vi "SoundGeneratorAD.vi"() -> ()   [LabVIEW 2019]
uses:
  <vilib>/sound2/lvsound2.llb/Sampling Mode.ctl
  <vilib>/sound2/lvsound2.llb/Sound Output Set Volume (Single).vi
  <vilib>/sound2/lvsound2.llb/Sound Output Write (DBL).vi
  <vilib>/measure/NI_MABase.lvlib
panel:
  in  "Stop":bool
  in  "Frequency Right":dbl(slide) scale=0.0..100.0
  in  "Amplitude Right":dbl(slide) scale=0.0..100.0
  in  "Frequency Left":dbl(slide) scale=0.0..100.0
  in  "Amplitude Left":dbl(slide) scale=0.0..100.0
  in  "# of samples":dbl
  in  "# of samples / ch":dbl
  in  "Volume":dbl(slide) scale=0.0..100.0
  in  "Output Device ID":dbl
  in  "Sound format":T1
  # "Default configurations for Sount format:\n\nSample rate: 44100 (Hz)\n# of channels: 2\nBits per sample: 16"
  # "How fast the sound\nis sampled per\nchannel"
  # "How fast the sound is sampled"
  # "Default: 0"
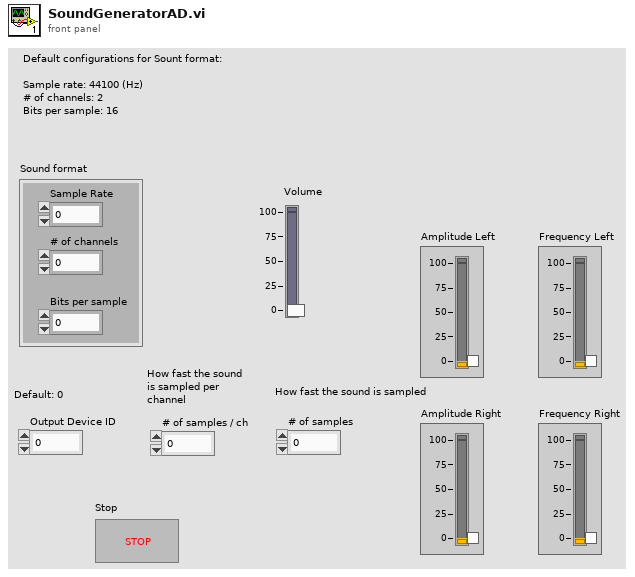
[diagram p1: front panel]
types:
  T1 = cluster{"Sample Rate":dbl, "# of channels":dbl, "Bits per sample":dbl}
  T2 = typedef "Sampling Mode.ctl" = i32
  T3 = typedef "Sound Output Task ID.ctl" = u32
  T4 = cluster{"# of samples / ch":dbl, "# of samples":dbl}
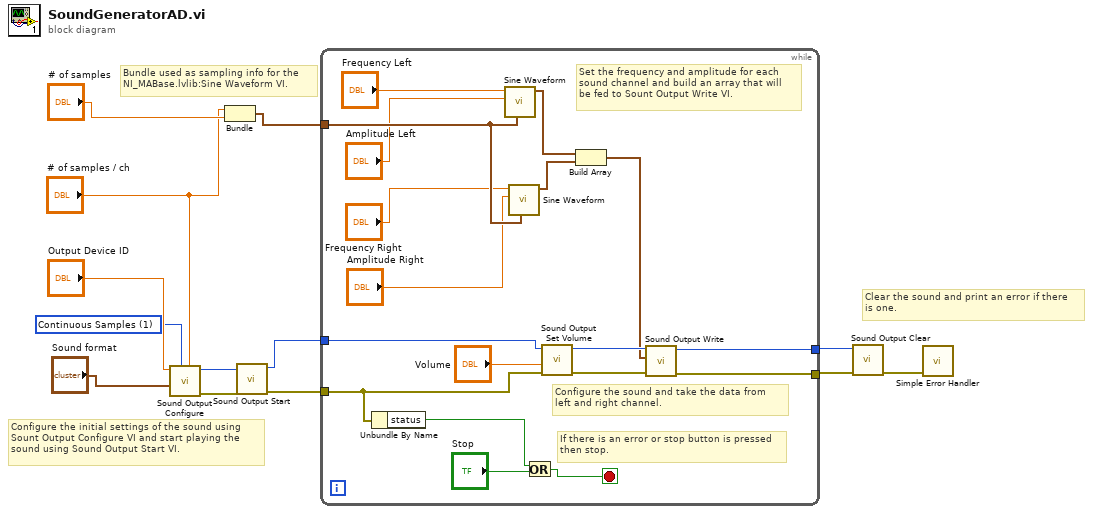
[diagram p0: block diagram]
diagram:
  w11 = T2 1 items=["Finite Samples", "Continuous Samples"] ("sample mode")
  # "Clear the sound and print an error if there\nis one."
  # "Bundle used as sampling info for the\nNI_MABase.lvlib:Sine Waveform VI."
  # "Configure the initial settings of the sound using\nSount Output Configure VI and start playing the\nsound using Sound Output Start VI."
  n1 = call <vilib>:"Sound Output Configure.vi"("number of samples/ch"="# of samples / ch", "sample mode"=w11, "sound format"="Sound format", "device ID"="Output Device ID") -> ("error out"=w10:errorcluster, "task ID"=w9:T3)  [unwired: 6 in]
  n2 = Bundle("# of samples / ch"="# of samples / ch", "# of samples"="# of samples") -> (w1:T4)  [unwired: 1 in]
  n3 = call <vilib>:"Sound Output Start.vi"("error in (no error)"=w10, "task ID"=w9) -> ("error out"=w6:errorcluster, "task ID out"=w5:T3)  [unwired: 8 in]
  n4 = while {
    tunnel: w6 -> [w28]
    tunnel: w5 -> [w26]
    tunnel: [w23] -> w4
    tunnel: [w22] -> w3
    tunnel: w1 -> [w21]
    stop <- w31 stop-if-true
    # "Set the frequency and amplitude for each\nsound channel and build an array that will\nbe fed to Sount Output Write VI."
    # "Configure the sound and take the data from\nleft and right channel."
    # "If there is an error or stop button is pressed\nthen stop."
    n5 = Unbundle By Name(w28) -> ("status"=w27:bool)
    n6 = call <vilib>:"Sine Waveform.vi"("sampling info"=w21, "amplitude"="Amplitude Left", "frequency"="Frequency Left") -> ("signal out"=w16:waveform(dbl))  [unwired: 7 in, 1 out]
    n7 = call <vilib>:"Sine Waveform.vi"("sampling info"=w21, "amplitude"="Amplitude Right", "frequency"="Frequency Right") -> ("signal out"=w15:waveform(dbl))  [unwired: 7 in, 1 out]
    n8 = Or(x=w27, y="Stop") -> (x .or. y?=w31:bool)
    n9 = call-poly <vilib>:"Sound Output Set Volume.vi"("error in (no error)"=w28, "volume"="Volume", "task ID"=w26) -> ("error out"=w25:errorcluster, "task ID out"=w24:T3)  [unwired: 7 in]
    n10 = Build Array(w16, w15) -> (w14:waveform(dbl)[])
    n11 = call-poly <vilib>:"Sound Output Write.vi"("error in (no error)"=w25, "data"=w14, "task ID"=w24) -> ("error out"=w22:errorcluster, "task ID out"=w23:T3)  [unwired: 7 in]
  }
  n12 = call <vilib>:"Sound Output Clear.vi"("error in (no error)"=w3, "task ID"=w4) -> ("error out"=w2:errorcluster)  [unwired: 9 in]
  n13 = call <vilib>:"Simple Error Handler.vi"("error in (no error)"=w2) -> ()  [unwired: 4 in, 5 out]
